vi "Destroy.vi"(0 "reference in":refnum<class "Gasoline Engine Factory.lvclass">, 11 "Error In":errorcluster) -> (4 "reference out":refnum<class "Gasoline Engine Factory.lvclass">, 15 "Error Out":errorcluster)   [LabVIEW 2024, in "Gasoline Engine Factory.lvclass"]
uses:
  Gasoline Engine Factory.lvclass
  Gasoline Engine Factory.lvclass/Gasoline Engine Factory.ctl
  EngineFactory/EngineFactory.lvclass
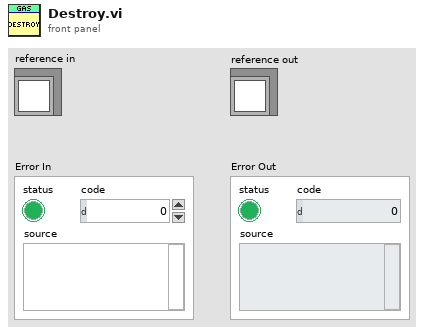
[diagram p1: front panel]
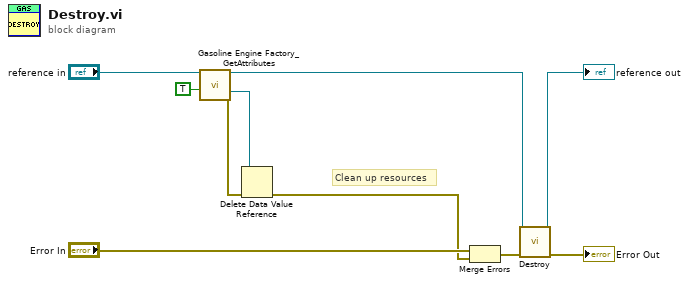
[diagram p0: block diagram]
diagram:
  # "Clean up resources"
  n1 = call "Gasoline Engine Factory_GetAttributes.vi"("reference in"="reference in", "OnlyGetDvrReference(False)"=TRUE) -> ("reference out"=w4:refnum<class "Gasoline Engine Factory.lvclass">, "DataRef"=w9:refnum<data-value>, "Error Out"=w10:errorcluster)  [unwired: 10 in, 1 out]
  n2 = Delete Data Value Reference(data value reference=w9, error in=w10) -> (error out=w7:errorcluster)  [unwired: 1 out]
  n3 = Merge Errors("Error In", w7) -> (w5:errorcluster)
  n4 = call-parent "Destroy.vi"("reference in"=w4, "Error In"=w5) -> ("reference out"=→"reference out":refnum<class "Gasoline Engine Factory.lvclass">, "Error Out"=→"Error Out":errorcluster)  [unwired: 12 in]
